vi "test_libssh2_session_callback_set.vi"() -> ()   [LabVIEW 2013, in "libssh2_integration_tests.lvlib"]
uses:
  libssh2_integration_tests.lvlib
  libssh2/libssh2_session_abstract.ctl
  libssh2/libssh2_session_callback_type.ctl
  libssh2/libssh2_init_default.vi
  libssh2/libssh2_session_handshake_tcp.vi
  libssh2/libssh2.lvlib
  <vilib>/addons/_JKI Toolkits/Caraya/classes/Test/Test.lvclass
  <vilib>/addons/_JKI Toolkits/Caraya/classes/Assert/Assert.lvclass
panel:
  out "error out":errorcluster
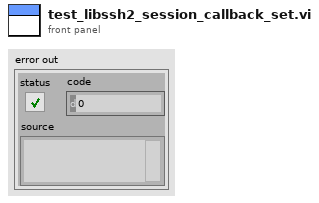
[diagram p1: front panel]
types:
  T1 = typedef "libssh2.lvlib/libssh2_session_abstract.ctl" = cluster{"send":refnum<vi>, "receive":refnum<vi>}
  T2 = typedef "libssh2.lvlib/Session Refnum.ctl" = refnum<k1>
  T3 = typedef "libssh2.lvlib/libssh2_session_callback_type.ctl" = enum16{"Ignore", "Debug", "Disconnect", "MAC Error", "X11", "Send", "Receive", "Auth Agent", "Auth Agent Identities", "Auth Agent Sign"}
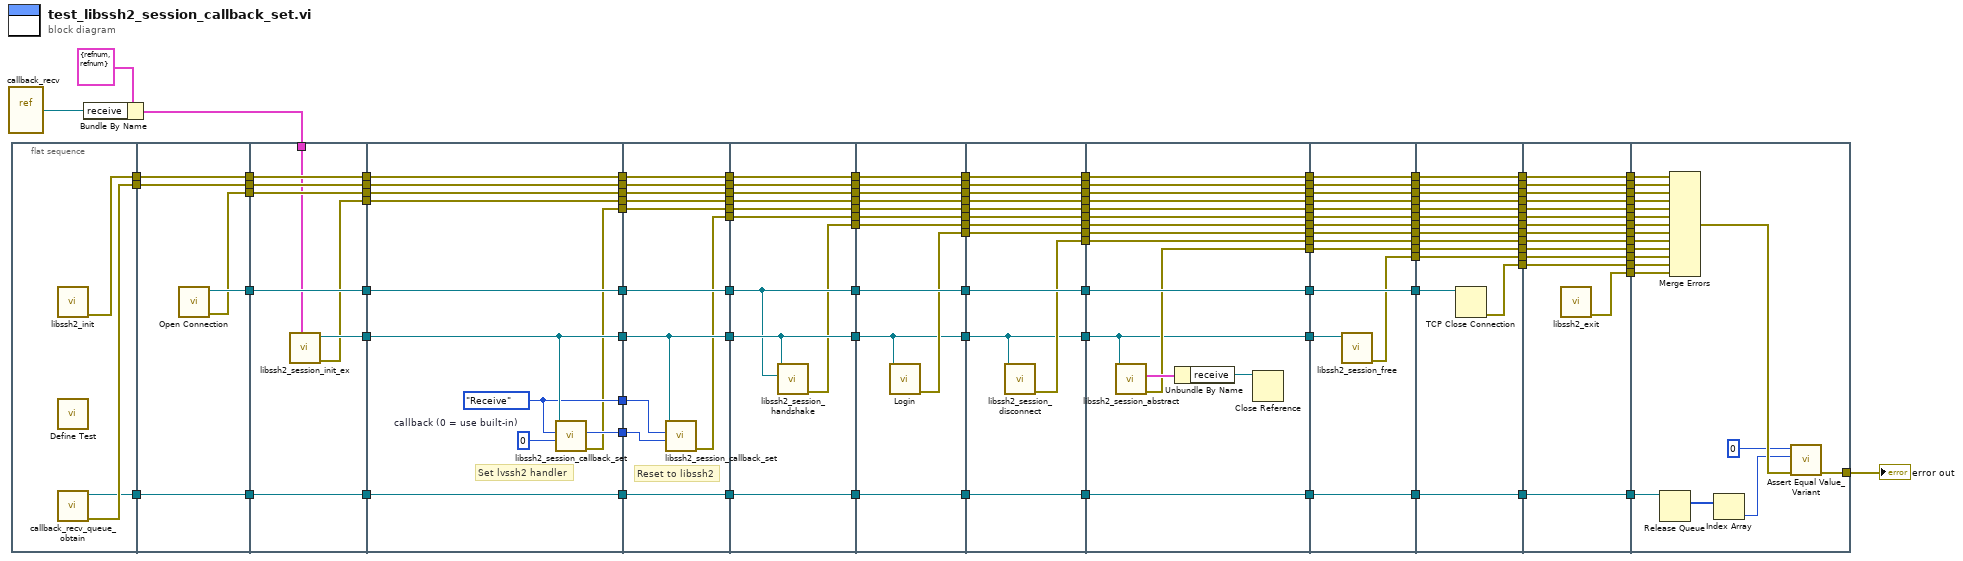
[diagram p0: block diagram]
diagram:
  n1 = vi-ref "callback_recv.vi"() -> (w123:refnum<vi>)
  n2 = flat-sequence {
    tunnel: [w127] -> w122
    tunnel: [w126] -> w105
    tunnel: [w125] -> w35
    tunnel: [w132] -> w121
    tunnel: w122 -> [w131]
    tunnel: [w131] -> w120
    tunnel: [w130] -> w119
    tunnel: w105 -> [w129]
    tunnel: [w129] -> w104
    tunnel: [w128] -> w36
    tunnel: w35 -> [w128]
    tunnel: w121 -> [w140]
    tunnel: [w140] -> w100
    tunnel: w120 -> [w139]
    tunnel: [w139] -> w99
    tunnel: w119 -> [w138]
    tunnel: [w138] -> w98
    tunnel: [w137] -> w97
    tunnel: [w136] -> w96
    tunnel: w104 -> [w135]
    tunnel: [w135] -> w95
    tunnel: w101 -> [w134]
    tunnel: [w133] -> w37
    tunnel: w36 -> [w133]
    tunnel: w100 -> [w151]
    tunnel: [w151] -> w33
    tunnel: w99 -> [w150]
    tunnel: [w150] -> w31
    tunnel: w98 -> [w149]
    tunnel: [w149] -> w29
    tunnel: w97 -> [w146]
    tunnel: [w146] -> w27
    tunnel: w96 -> [w148]
    tunnel: [w148] -> w25
    tunnel: w95 -> [w147]
    tunnel: [w147] -> w23
    tunnel: w37 -> [w145]
    tunnel: [w145] -> w21
    tunnel: [w144] -> w19
    tunnel: [w143] -> w18
    tunnel: [w142] -> w17
    tunnel: w33 -> [w162]
    tunnel: [w162] -> w32
    tunnel: w31 -> [w161]
    tunnel: [w161] -> w30
    tunnel: w29 -> [w160]
    tunnel: [w160] -> w28
    tunnel: w27 -> [w154]
    tunnel: [w154] -> w26
    tunnel: w25 -> [w159]
    tunnel: [w159] -> w24
    tunnel: w23 -> [w158]
    tunnel: [w158] -> w22
    tunnel: w21 -> [w157]
    tunnel: [w157] -> w20
    tunnel: w19 -> [w156]
    tunnel: w18 -> [w155]
    tunnel: w17 -> [w153]
    tunnel: [w153] -> w16
    tunnel: [w152] -> w8
    tunnel: w32 -> [w168]
    tunnel: [w168] -> w94
    tunnel: w30 -> [w172]
    tunnel: [w172] -> w93
    tunnel: w28 -> [w171]
    tunnel: [w171] -> w92
    tunnel: [w170] -> w91
    tunnel: w26 -> [w170]
    tunnel: w24 -> [w169]
    tunnel: [w169] -> w90
    tunnel: [w167] -> w89
    tunnel: w22 -> [w166]
    tunnel: [w166] -> w88
    tunnel: [w165] -> w38
    tunnel: w20 -> [w165]
    tunnel: w16 -> [w164]
    tunnel: [w164] -> w15
    tunnel: w8 -> [w163]
    tunnel: [w163] -> w7
    tunnel: w94 -> [w183]
    tunnel: [w183] -> w52
    tunnel: w93 -> [w182]
    tunnel: [w182] -> w51
    tunnel: w92 -> [w181]
    tunnel: [w181] -> w50
    tunnel: w91 -> [w176]
    tunnel: w90 -> [w180]
    tunnel: [w180] -> w49
    tunnel: w89 -> [w179]
    tunnel: [w179] -> w48
    tunnel: w88 -> [w178]
    tunnel: [w178] -> w47
    tunnel: [w177] -> w46
    tunnel: [w176] -> w45
    tunnel: [w175] -> w39
    tunnel: w38 -> [w175]
    tunnel: w15 -> [w174]
    tunnel: [w174] -> w14
    tunnel: w7 -> [w173]
    tunnel: [w173] -> w6
    tunnel: w52 -> [w195]
    tunnel: [w195] -> w85
    tunnel: w51 -> [w194]
    tunnel: [w194] -> w84
    tunnel: w50 -> [w193]
    tunnel: [w193] -> w83
    tunnel: w49 -> [w192]
    tunnel: [w192] -> w82
    tunnel: [w191] -> w81
    tunnel: w48 -> [w190]
    tunnel: [w190] -> w80
    tunnel: w47 -> [w189]
    tunnel: [w189] -> w79
    tunnel: w46 -> [w188]
    tunnel: [w188] -> w78
    tunnel: [w187] -> w77
    tunnel: w45 -> [w187]
    tunnel: [w186] -> w40
    tunnel: w39 -> [w186]
    tunnel: w14 -> [w185]
    tunnel: [w185] -> w13
    tunnel: w6 -> [w184]
    tunnel: [w184] -> w5
    tunnel: w85 -> [w210]
    tunnel: [w210] -> w74
    tunnel: w84 -> [w209]
    tunnel: [w209] -> w72
    tunnel: w83 -> [w208]
    tunnel: [w208] -> w70
    tunnel: w82 -> [w207]
    tunnel: [w207] -> w68
    tunnel: w81 -> [w206]
    tunnel: [w206] -> w66
    tunnel: w80 -> [w205]
    tunnel: [w205] -> w64
    tunnel: w79 -> [w204]
    tunnel: [w204] -> w62
    tunnel: w78 -> [w203]
    tunnel: [w203] -> w60
    tunnel: w77 -> [w199]
    tunnel: [w200] -> w58
    tunnel: [w199] -> w56
    tunnel: [w198] -> w41
    tunnel: w40 -> [w198]
    tunnel: w13 -> [w197]
    tunnel: [w197] -> w12
    tunnel: w5 -> [w196]
    tunnel: [w196] -> w4
    tunnel: w74 -> [w224]
    tunnel: [w224] -> w73
    tunnel: w72 -> [w223]
    tunnel: [w223] -> w71
    tunnel: w70 -> [w222]
    tunnel: [w222] -> w69
    tunnel: w68 -> [w221]
    tunnel: [w221] -> w67
    tunnel: w66 -> [w220]
    tunnel: [w220] -> w65
    tunnel: w64 -> [w219]
    tunnel: [w219] -> w63
    tunnel: w62 -> [w218]
    tunnel: [w218] -> w61
    tunnel: w60 -> [w217]
    tunnel: [w217] -> w59
    tunnel: w58 -> [w216]
    tunnel: [w216] -> w57
    tunnel: w56 -> [w215]
    tunnel: [w214] -> w53
    tunnel: [w213] -> w42
    tunnel: w41 -> [w213]
    tunnel: w12 -> [w212]
    tunnel: [w212] -> w11
    tunnel: w4 -> [w211]
    tunnel: [w211] -> w3
    tunnel: w73 -> [w238]
    tunnel: w71 -> [w237]
    tunnel: [w237] -> w118
    tunnel: w69 -> [w236]
    tunnel: [w236] -> w117
    tunnel: [w235] -> w116
    tunnel: w67 -> [w234]
    tunnel: [w234] -> w115
    tunnel: w65 -> [w233]
    tunnel: [w233] -> w114
    tunnel: w63 -> [w232]
    tunnel: [w232] -> w113
    tunnel: w61 -> [w231]
    tunnel: [w231] -> w103
    tunnel: w59 -> [w230]
    tunnel: [w230] -> w87
    tunnel: w57 -> [w229]
    tunnel: [w229] -> w76
    tunnel: [w228] -> w54
    tunnel: w53 -> [w228]
    tunnel: [w227] -> w43
    tunnel: w42 -> [w227]
    tunnel: w11 -> [w226]
    tunnel: [w226] -> w10
    tunnel: w3 -> [w225]
    tunnel: [w225] -> w2
    tunnel: w118 -> [w252]
    tunnel: [w252] -> w112
    tunnel: w117 -> [w251]
    tunnel: [w251] -> w111
    tunnel: w116 -> [w250]
    tunnel: [w250] -> w110
    tunnel: [w249] -> w109
    tunnel: w115 -> [w248]
    tunnel: [w248] -> w108
    tunnel: w114 -> [w247]
    tunnel: [w247] -> w107
    tunnel: w113 -> [w246]
    tunnel: [w246] -> w106
    tunnel: w103 -> [w245]
    tunnel: [w245] -> w102
    tunnel: w87 -> [w244]
    tunnel: [w244] -> w86
    tunnel: w76 -> [w243]
    tunnel: [w243] -> w75
    tunnel: [w242] -> w55
    tunnel: w54 -> [w242]
    tunnel: [w241] -> w44
    tunnel: w43 -> [w241]
    tunnel: w10 -> [w240]
    tunnel: [w240] -> w9
    tunnel: w2 -> [w239]
    tunnel: [w239] -> w1
    tunnel: w112 -> [w271]
    tunnel: w111 -> [w270]
    tunnel: w110 -> [w269]
    tunnel: w109 -> [w268]
    tunnel: w108 -> [w267]
    tunnel: w107 -> [w266]
    tunnel: [w264] -> w34
    tunnel: w106 -> [w263]
    tunnel: w102 -> [w262]
    tunnel: w86 -> [w261]
    tunnel: w75 -> [w260]
    tunnel: w55 -> [w259]
    tunnel: w44 -> [w258]
    tunnel: w9 -> [w257]
    tunnel: w1 -> [w256]
    frame #0 {
      n3 = call-poly "libssh2_init.vi"() -> ("error out"=w127:errorcluster)  [unwired: 11 in]
      n4 = call <vilib>:"Define Test.vi"() -> ()  [unwired: 10 in, 2 out]
      n5 = call "callback_recv_queue_obtain.vi"() -> ("error out"=w126:errorcluster, "queue out"=w125:refnum<queue>)  [unwired: 10 in]
    }
    frame #1 {
      n6 = call "Open Connection.vi"() -> ("error out"=w130:errorcluster, "connection ID"=w132:refnum<k5>)  [unwired: 10 in]
    }
    frame #2 {
      n7 = call "libssh2_session_init_ex.vi"("abstract"=w134) -> ("error out"=w136:errorcluster, "session"=w137:T2)  [unwired: 9 in]
    }
    frame #3 {
      w141 = u64 0  # callback (0 = use built-in)
      w144 = libssh2_session_callback_type."Receive" ("callback type")
      # "Set lvssh2 handler"
      n8 = call "libssh2_session_callback_set.vi"("callback (0 = use built-in)"=w141, "callback type"=w144, "session"=w146) -> ("error out"=w142:errorcluster, "previous callback"=w143:u64)  [unwired: 7 in]
    }
    frame #4 {
      # "Reset to libssh2"
      n9 = call "libssh2_session_callback_set.vi"("callback (0 = use built-in)"=w155, "callback type"=w156, "session"=w154) -> ("error out"=w152:errorcluster)  [unwired: 7 in, 1 out]
    }
    frame #5 {
      n10 = call-poly "libssh2_session_handshake.vi"("tcp connection"=w168, "session"=w170) -> ("error out"=w167:errorcluster)  [unwired: 9 in]
    }
    frame #6 {
      n11 = call "Login.vi"("session"=w176) -> ("error out"=w177:errorcluster)  [unwired: 10 in]
    }
    frame #7 {
      n12 = call "libssh2_session_disconnect.vi"("session"=w187) -> ("error out"=w191:errorcluster)  [unwired: 10 in]
    }
    frame #8 {
      n13 = call "libssh2_session_abstract.vi"("session"=w199) -> ("error out"=w200:errorcluster, "abstract"=w202:T1)  [unwired: 9 in]
      n14 = Unbundle By Name(w202) -> ("receive"=w201:refnum<vi>)
      n15 = Close Reference(reference=w201) -> ()  [unwired: 1 in, 1 out]
    }
    frame #9 {
      n16 = call "libssh2_session_free.vi"("session"=w215) -> ("error out"=w214:errorcluster)  [unwired: 10 in]
    }
    frame #10 {
      n17 = TCP Close Connection(connection ID=w238) -> (error out=w235:errorcluster)  [unwired: 2 in, 1 out]
    }
    frame #11 {
      n18 = call "libssh2_exit.vi"() -> ("error out"=w249:errorcluster)  [unwired: 11 in]
    }
    frame #12 {
      n19 = Release Queue(queue=w258) -> (remaining elements=w255:i32[])  [unwired: 2 in, 2 out]
      n20 = Merge Errors(w271, w262, w270, w267, w257, w256, w263, w261, w266, w260, w259, w269, w268) -> (w265:errorcluster)
      n21 = Index Array(array=w255) -> (element=w254:i32)  [unwired: 1 in]
      n22 = call <vilib>:"Assert Equal Value_Variant.vi"("error in (no error)"=w265, "Y"=w254, "X"=0 ("element")) -> ("error out"=w264:errorcluster)  [unwired: 7 in, 1 out]
    }
  }
  n23 = Bundle By Name(cluster=T1 {"send"=refnum, "receive"=refnum} ("abstract"), "receive"=w123) -> (w101:T1)
  "error out" <- w34
